vi "FT10_Semi-Auto Power Set and Read.vi"(10 "Auto Set Power Cluster in":T1 {"Power Level" format="%.1f"}, 11 "Message Handling Cluster in":T5={"Fornax Connected?"=refnum, "Unitherm Connected?"=refnum, "M4X Connected?"=refnum, "Unitherm Connect/Disconnect"=refnum, "Fornax Connection"=refnum, "UNITHERM Connection"="", "M4X Connection"=0, "FPGA VI Reference Out"=refnum, "PXI-7854R Connected?"=refnum, "Fornax Connect/Disconnect"=refnum, "7854 Connect/Disconnect"=refnum, "M4X Connect/Disconnect"=refnum, "Config cluster"={"Unitherm Port"="COM4", "Simulate Values"=TRUE, "Fornax Connect Attempts"=0}, "Log Queue"=refnum, "Log Analysis Cluster - Current"={"RMS"=0.0, "Envelope Frequency"=0.0, "Peak"=0.0, "Crest Factor"=0.0, "Duty Cyle %"=0.0, "P-P"=0.0, "Frequency"=0.0, "THD"=0.0, "Postive Peak"=0.0, "Negative Peak"=0.0, "Mag_H1"=0.0, "Phase_H1"=0.0, "Mag_H3"=0.0, "Phase_H3"=0.0, "Mag_H5"=0.0, "Phase_H5"=0.0}, "Log Waveform Cluster - Current"={"t0"=timestamp(0 s since 1904-01-01), "dt"=1.0, "Y"=[]}, "Log Time"=timestamp(0 s since 1904-01-01), "Log Flag"=FALSE, "Log - Activation Settings Cluster"={"Log - Unitherm Load"="", "Log - Port"="", "Log - Mode"="", "Log - Power Level"=""}, "Log - Port Mode Cluster"={"Mono1 Cut Enum"=enum."Pure", "Mono2 Cut Enum"=enum."Pure", "Mono1 Coag Enum"=enum."Spray", "Mono2 Coag Enum"=enum."Spray", "Bipolar Enum"=enum."Standard"}, "Log Analysis Cluster - Diff Voltage"={"RMS"=0.0, "Envelope Frequency"=0.0, "Peak"=0.0, "Crest Factor"=0.0, "Duty Cyle %"=0.0, "P-P"=0.0, "Frequency"=0.0, "THD"=0.0, "Postive Peak"=0.0, "Negative Peak"=0.0, "Mag_H1"=0.0, "Phase_H1"=0.0, "Mag_H3"=0.0, "Phase_H3"=0.0, "Mag_H5"=0.0, "Phase_H5"=0.0}, "Log Waveform Cluster - Diff Voltage"={"t0"=timestamp(0 s since 1904-01-01), "dt"=1.0, "Y"=[]}, "Indicator Cluster"={"Mono1 - Cut Power"=refnum, "Mono1 - Coag Power"=refnum, "Mono2 - Cut Power"=refnum, "Mono2 - Coag Power"=refnum, "Bipolar Power"=refnum, "Mono1 Cut Enum"=refnum, "Mono1 Coag Enum"=refnum, "Mono2 Cut Enum"=refnum, "Mono2 Coag Enum"=refnum, "Bipolar Enum"=refnum}, "Log Power Level Cluster"={"Log Mono1 Cut Power"="", "Log Mono1 Coag Power"="", "Log Mono2 Cut Power"="", "Log Mono2 Coag Power"="", "Log Bipolar Power"=""}, "Footswitch Cluster"={"PXI-2565 reset device (boolean value)"=TRUE, "topology name"="2565/16-SPST", "PXI-2565 simulate (boolean value)"=FALSE, "PXI-2565 resource name"=""}}) -> (2 "Auto Set Power Cluster out":T1 {"Power Level" format="%.1f"}, 3 "Message Handling Cluster out":T5={"Fornax Connected?"=refnum, "Unitherm Connected?"=refnum, "M4X Connected?"=refnum, "Unitherm Connect/Disconnect"=refnum, "Fornax Connection"=refnum, "UNITHERM Connection"="", "M4X Connection"=0, "FPGA VI Reference Out"=refnum, "PXI-7854R Connected?"=refnum, "Fornax Connect/Disconnect"=refnum, "7854 Connect/Disconnect"=refnum, "M4X Connect/Disconnect"=refnum, "Config cluster"={"Unitherm Port"="COM4", "Simulate Values"=TRUE, "Fornax Connect Attempts"=0}, "Log Queue"=refnum, "Log Analysis Cluster - Current"={"RMS"=0.0, "Envelope Frequency"=0.0, "Peak"=0.0, "Crest Factor"=0.0, "Duty Cyle %"=0.0, "P-P"=0.0, "Frequency"=0.0, "THD"=0.0, "Postive Peak"=0.0, "Negative Peak"=0.0, "Mag_H1"=0.0, "Phase_H1"=0.0, "Mag_H3"=0.0, "Phase_H3"=0.0, "Mag_H5"=0.0, "Phase_H5"=0.0}, "Log Waveform Cluster - Current"={"t0"=timestamp(0 s since 1904-01-01), "dt"=1.0, "Y"=[]}, "Log Time"=timestamp(0 s since 1904-01-01), "Log Flag"=FALSE, "Log - Activation Settings Cluster"={"Log - Unitherm Load"="", "Log - Port"="", "Log - Mode"="", "Log - Power Level"=""}, "Log - Port Mode Cluster"={"Mono1 Cut Enum"=enum."Pure", "Mono2 Cut Enum"=enum."Pure", "Mono1 Coag Enum"=enum."Spray", "Mono2 Coag Enum"=enum."Spray", "Bipolar Enum"=enum."Standard"}, "Log Analysis Cluster - Diff Voltage"={"RMS"=0.0, "Envelope Frequency"=0.0, "Peak"=0.0, "Crest Factor"=0.0, "Duty Cyle %"=0.0, "P-P"=0.0, "Frequency"=0.0, "THD"=0.0, "Postive Peak"=0.0, "Negative Peak"=0.0, "Mag_H1"=0.0, "Phase_H1"=0.0, "Mag_H3"=0.0, "Phase_H3"=0.0, "Mag_H5"=0.0, "Phase_H5"=0.0}, "Log Waveform Cluster - Diff Voltage"={"t0"=timestamp(0 s since 1904-01-01), "dt"=1.0, "Y"=[]}, "Indicator Cluster"={"Mono1 - Cut Power"=refnum, "Mono1 - Coag Power"=refnum, "Mono2 - Cut Power"=refnum, "Mono2 - Coag Power"=refnum, "Bipolar Power"=refnum, "Mono1 Cut Enum"=refnum, "Mono1 Coag Enum"=refnum, "Mono2 Cut Enum"=refnum, "Mono2 Coag Enum"=refnum, "Bipolar Enum"=refnum}, "Log Power Level Cluster"={"Log Mono1 Cut Power"="", "Log Mono1 Coag Power"="", "Log Mono2 Cut Power"="", "Log Mono2 Coag Power"="", "Log Bipolar Power"=""}, "Footswitch Cluster"={"PXI-2565 reset device (boolean value)"=TRUE, "topology name"="2565/16-SPST", "PXI-2565 simulate (boolean value)"=FALSE, "PXI-2565 resource name"=""}})   [LabVIEW 2024]
uses:
  Controls/Control_Message Handling Cluster.ctl
  Controls/Control_M4X Connection.ctl
  Controls/Control_PXI-7854R FPGA Reference.ctl
  Controls/Control_Config Cluster.ctl
  Controls/Control_Config Unitherm Port.ctl
  Controls/Control_Config Simulate Values.ctl
  Controls/Control_Config Fornax Connect Attempts.ctl
  Controls/Control_Log Queue.ctl
  Controls/Control_Log Cluster.ctl
  Controls/Control_Log Time.ctl
  Controls/Control_Log Waveform Cluster - Current.ctl
  Controls/Control_Log Analysis Cluster - Current.ctl
  Controls/Control_Log Activation Settings Cluster.ctl
  Controls/Control_Log Unitherm Load.ctl
  Controls/Control_Log Port.ctl
  Controls/Control_Log Mode.ctl
  Controls/Control_Log Power Level.ctl
  Controls/Control_Log Waveform Cluster - Diff Voltage.ctl
  Controls/Control_Log Analysis Cluster - Diff Voltage.ctl
  Controls/Control_Log Flag.ctl
  Controls/Control_Log Port Mode Cluster.ctl
  Controls/Control_Fornax Mono1 Cut Enum.ctl
  Controls/Control_Fornax Mono2 Cut Enum.ctl
  Controls/Control_Fornax Mono1 Coag Enum.ctl
  Controls/Control_Fornax Mono2 Coag Enum.ctl
  Controls/Control_Fornax Bipolar Enum.ctl
  Controls/Control_Indicator Cluster.ctl
  Controls/Control_Log Power Level Cluster.ctl
  Controls/Control_Log Mono1 Cut Power.ctl
  Controls/Control_Log Mono1 Coag Power.ctl
  Controls/Control_Log Mono2 Cut Power.ctl
  Controls/Control_Log Mono2 Coag Power.ctl
  Controls/Control_Log Bipolar Power.ctl
  Controls/Control_Footswitch Reset Device Bool.ctl
  <instrlib>/niSwitch/niSwitch.llb/niSwitch Topologies.ctl
  Controls/Control_Footswitch Simulate Bool.ctl
  Controls/Control_Footswitch Resource Name.ctl
  Controls/Control_Auto Set Power Cluster.ctl
  Controls/Control_Semi-Auto Port.ctl
  Controls/Control_Semi-Auto Mode.ctl
  Controls/Control_Semi-Auto Power Level.ctl
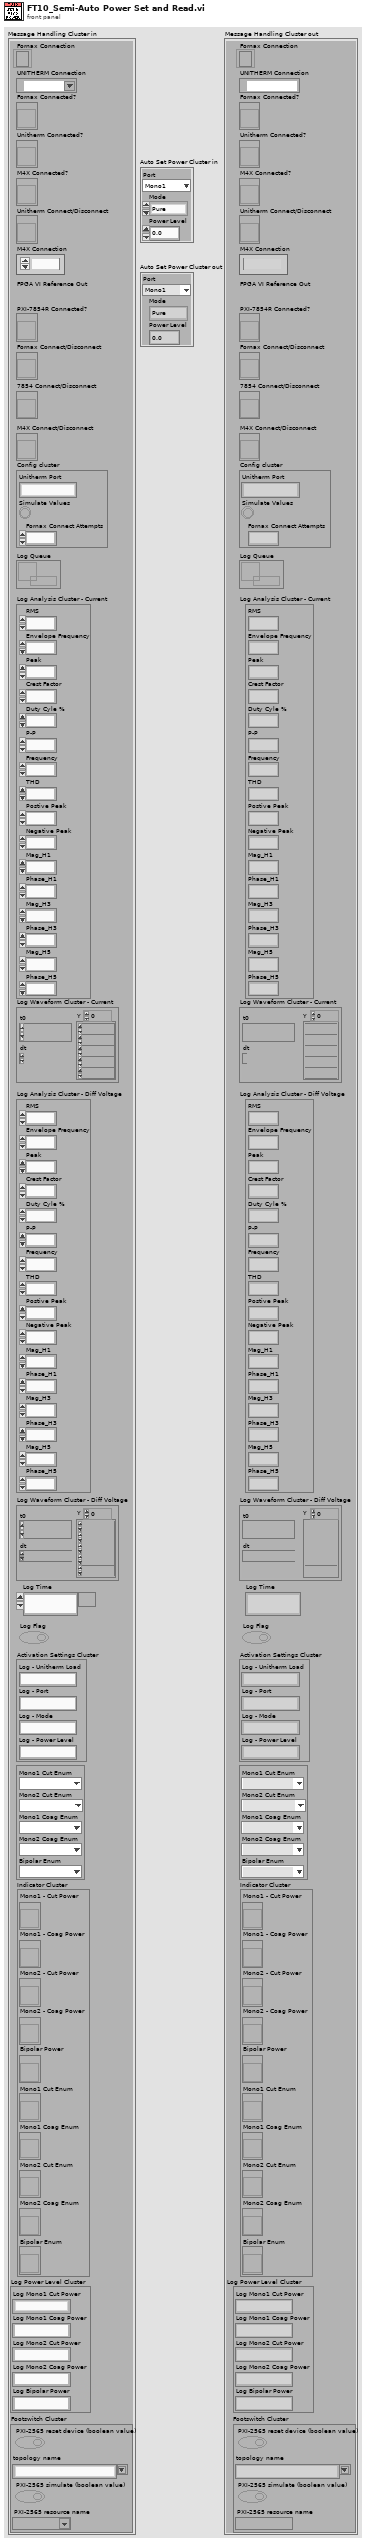
[diagram p1: front panel]
types:
  T1 = typedef "Control_Auto Set Power Cluster.ctl" = cluster{"Port":T2, "Mode":T3, "Power Level":T4}
  T2 = typedef "Control_Semi-Auto Port.ctl" = enum16{"Mono1", "Mono2", "Bipolar", "Ligasure", "Error"}
  T3 = typedef "Control_Semi-Auto Mode.ctl" = enum16{"Pure", "Blend", "Spray", "Fulgerate", "Standard", "Macro", "Precision", "Ligasure", "Error"}
  T4 = typedef "Control_Semi-Auto Power Level.ctl" = dbl
  T5 = typedef "Control_Message Handling Cluster.ctl" = cluster{"Fornax Connected?":refnum<vi>, "Unitherm Connected?":refnum<vi>, "M4X Connected?":refnum<vi>, "Unitherm Connect/Disconnect":refnum<vi>, "Fornax Connection":refnum<k5>, "UNITHERM Connection":refnum<visa-resource-name>, "M4X Connection":T6, "FPGA VI Reference Out":T7, "PXI-7854R Connected?":refnum<vi>, "Fornax Connect/Disconnect":refnum<vi>, "7854 Connect/Disconnect":refnum<vi>, "M4X Connect/Disconnect":refnum<vi>, "Config cluster":T8, "Log Queue":T12, "Log Analysis Cluster - Current":T13, "Log Waveform Cluster - Current":T14, "Log Time":T15, "Log Flag":T16, "Log - Activation Settings Cluster":T17, "Log - Port Mode Cluster":T22, "Log Analysis Cluster - Diff Voltage":T28, "Log Waveform Cluster - Diff Voltage":T29, "Indicator Cluster":T30, "Log Power Level Cluster":T31, "Footswitch Cluster":cluster{"PXI-2565 reset device (boolean value)":T37, "topology name":T38, "PXI-2565 simulate (boolean value)":T39, "PXI-2565 resource name":T40}}
  T6 = typedef "Control_M4X Connection.ctl" = u32
  T7 = typedef "Control_PXI-7854R FPGA Reference.ctl" = refnum<k20>
  T8 = typedef "Control_Config Cluster.ctl" = cluster{"Unitherm Port":T9, "Simulate Values":T10, "Fornax Connect Attempts":T11}
  T9 = typedef "Control_Config Unitherm Port.ctl" = string
  T10 = typedef "Control_Config Simulate Values.ctl" = bool
  T11 = typedef "Control_Config Fornax Connect Attempts.ctl" = i32
  T12 = typedef "Control_Log Queue.ctl" = refnum<queue>
  T13 = typedef "Control_Log Analysis Cluster - Current.ctl" = cluster{"RMS":dbl, "Envelope Frequency":dbl, "Peak":dbl, "Crest Factor":dbl, "Duty Cyle %":dbl, "P-P":dbl, "Frequency":dbl, "THD":dbl, "Postive Peak":dbl, "Negative Peak":dbl, "Mag_H1":dbl, "Phase_H1":dbl, "Mag_H3":dbl, "Phase_H3":dbl, "Mag_H5":dbl, "Phase_H5":dbl}
  T14 = typedef "Control_Log Waveform Cluster - Current.ctl" = waveform(dbl)
  T15 = typedef "Control_Log Time.ctl" = timestamp
  T16 = typedef "Control_Log Flag.ctl" = bool
  T17 = typedef "Control_Log Activation Settings Cluster.ctl" = cluster{"Log - Unitherm Load":T18, "Log - Port":T19, "Log - Mode":T20, "Log - Power Level":T21}
  T18 = typedef "Control_Log Unitherm Load.ctl" = string
  T19 = typedef "Control_Log Port.ctl" = string
  T20 = typedef "Control_Log Mode.ctl" = string
  T21 = typedef "Control_Log Power Level.ctl" = string
  T22 = typedef "Control_Log Port Mode Cluster.ctl" = cluster{"Mono1 Cut Enum":T23, "Mono2 Cut Enum":T24, "Mono1 Coag Enum":T25, "Mono2 Coag Enum":T26, "Bipolar Enum":T27}
  T23 = typedef "Control_Fornax Mono1 Cut Enum.ctl" = enum16{"Pure", "Blend"}
  T24 = typedef "Control_Fornax Mono2 Cut Enum.ctl" = enum16{"Pure", "Blend"}
  T25 = typedef "Control_Fornax Mono1 Coag Enum.ctl" = enum16{"Fulgerate", "Spray"}
  T26 = typedef "Control_Fornax Mono2 Coag Enum.ctl" = enum16{"Fulgerate", "Spray"}
  T27 = typedef "Control_Fornax Bipolar Enum.ctl" = enum16{"Standard", "Macro", "Precision"}
  T28 = typedef "Control_Log Analysis Cluster - Diff Voltage.ctl" = cluster{"RMS":dbl, "Envelope Frequency":dbl, "Peak":dbl, "Crest Factor":dbl, "Duty Cyle %":dbl, "P-P":dbl, "Frequency":dbl, "THD":dbl, "Postive Peak":dbl, "Negative Peak":dbl, "Mag_H1":dbl, "Phase_H1":dbl, "Mag_H3":dbl, "Phase_H3":dbl, "Mag_H5":dbl, "Phase_H5":dbl}
  T29 = typedef "Control_Log Waveform Cluster - Diff Voltage.ctl" = waveform(dbl)
  T30 = typedef "Control_Indicator Cluster.ctl" = cluster{"Mono1 - Cut Power":refnum<vi>, "Mono1 - Coag Power":refnum<vi>, "Mono2 - Cut Power":refnum<vi>, "Mono2 - Coag Power":refnum<vi>, "Bipolar Power":refnum<vi>, "Mono1 Cut Enum":refnum<vi>, "Mono1 Coag Enum":refnum<vi>, "Mono2 Cut Enum":refnum<vi>, "Mono2 Coag Enum":refnum<vi>, "Bipolar Enum":refnum<vi>}
  T31 = typedef "Control_Log Power Level Cluster.ctl" = cluster{"Log Mono1 Cut Power":T32, "Log Mono1 Coag Power":T33, "Log Mono2 Cut Power":T34, "Log Mono2 Coag Power":T35, "Log Bipolar Power":T36}
  T32 = typedef "Control_Log Mono1 Cut Power.ctl" = string
  T33 = typedef "Control_Log Mono1 Coag Power.ctl" = string
  T34 = typedef "Control_Log Mono2 Cut Power.ctl" = string
  T35 = typedef "Control_Log Mono2 Coag Power.ctl" = string
  T36 = typedef "Control_Log Bipolar Power.ctl" = string
  T37 = typedef "Control_Footswitch Reset Device Bool.ctl" = bool
  T38 = typedef "niSwitch Topologies.ctl" = string
  T39 = typedef "Control_Footswitch Simulate Bool.ctl" = bool
  T40 = typedef "Control_Footswitch Resource Name.ctl" = refnum<k15>
  T41 = typedef "Control_Semi-Auto Power Level - For Loop Iterations.ctl" = i32
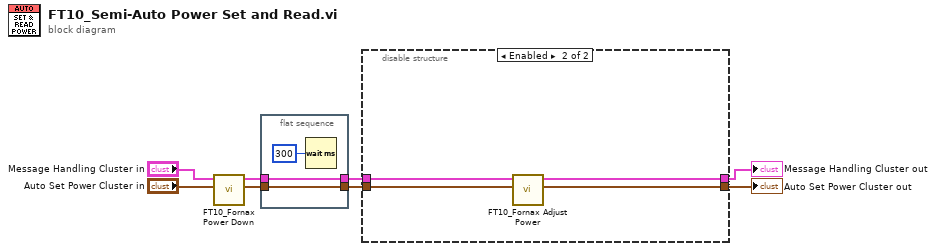
[diagram p0: block diagram]
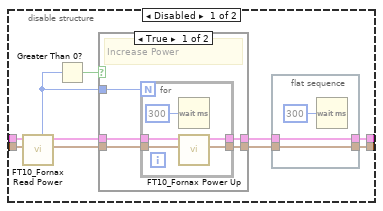
[diagram p2: hidden frame]
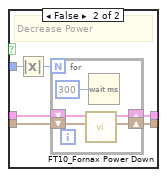
[diagram p3: hidden frame]
diagram:
  n1 = call "FT10_Fornax Power Down.vi"("Auto Set Power Cluster in"="Auto Set Power Cluster in", "Message Handling Cluster in"="Message Handling Cluster in") -> ("Auto Set Power Cluster out"=w3:T1, "Message Handling Cluster out"=w5:T5)  [unwired: 8 in]
  n2 = flat-sequence {
    tunnel: [w10] -> w6
    tunnel: w5 -> [w10]
    tunnel: [w9] -> w4
    tunnel: w3 -> [w9]
    frame #0 {
      n3 = Wait (ms)(milliseconds to wait=u32 300) -> ()  [unwired: 1 out]
    }
  }
  n4 = disable-structure shown="Enabled" {
    disable-tunnel: w6 -> [w17 w49]
    disable-tunnel: w4 -> [w16 w48]
    disable-tunnel: [w15 w46] -> w2
    disable-tunnel: [w12 w47] -> w1
    frame Disabled {
      n5 = call "FT10_Fornax Read Power.vi"("Auto Set Power Cluster in"=w16, "Message Handling Cluster in"=w17) -> ("Auto Set Power Cluster out"=w18:T1, "Message Handling Cluster out"=w19:T5, "For Loop Iterations"=w20:T41)  [unwired: 7 in]
      n6 = Greater Than 0?(x=w20) -> (x > 0?=w21:bool)
      n7 = case shown="True" w21 {
        tunnel: w20 -> [w29 w40]
        tunnel: w19 -> [w28 w39]
        tunnel: w18 -> [w27 w38]
        tunnel: [w26 w36] -> w13
        tunnel: [w25 w35] -> w14
        frame True {
          # "Increase Power"
          n8 = for {
            N: w29 -> [_]
            tunnel: w28 -> [w34]
            tunnel: w27 -> [w33]
            tunnel: [w32] -> w26
            tunnel: [w31] -> w25
            n9 = Wait (ms)(milliseconds to wait=u32 300) -> ()  [unwired: 1 out]
            n10 = call "FT10_Fornax Power Up.vi"("Auto Set Power Cluster in"=w33, "Message Handling Cluster in"=w34) -> ("Auto Set Power Cluster out"=w31:T1, "Message Handling Cluster out"=w32:T5)  [unwired: 8 in]
          }
        }
        frame False {
          # "Decrease Power"
          n11 = Absolute Value(x=w40) -> (abs(x)=w37:T41)
          n12 = for {
            N: w37 -> [_]
            shift-right: [w43] -> w36
            shift-left: w39 -> [w45]
            shift-right: [w42] -> w35
            shift-left: w38 -> [w44]
            n13 = call "FT10_Fornax Power Down.vi"("Auto Set Power Cluster in"=w44, "Message Handling Cluster in"=w45) -> ("Auto Set Power Cluster out"=w42:T1, "Message Handling Cluster out"=w43:T5)  [unwired: 8 in]
            n14 = Wait (ms)(milliseconds to wait=u32 300) -> ()  [unwired: 1 out]
          }
        }
      }
      n15 = flat-sequence {
        tunnel: [w23] -> w12
        tunnel: w13 -> [w23]
        tunnel: [w22] -> w15
        tunnel: w14 -> [w22]
        frame #0 {
          n16 = Wait (ms)(milliseconds to wait=u32 300) -> ()  [unwired: 1 out]
        }
      }
    }
    frame Enabled {
      n17 = call "FT10_Fornax Adjust Power.vi"("Auto Set Power Cluster in"=w48, "Message Handling Cluster in"=w49) -> ("Auto Set Power Cluster out"=w46:T1, "Message Handling Cluster out"=w47:T5)  [unwired: 8 in]
    }
  }
  "Message Handling Cluster out" <- w1
  "Auto Set Power Cluster out" <- w2
